vi "PC Code for Music Player.vi"() -> ()   [LabVIEW 2014]
uses:
  <vilib>/Utility/file.llb/Read From Spreadsheet File (I64).vi
panel:
  in  "stop":bool
  out "Debug Durations":i32[](array[numeric])
  out "Debug Notes":i32[](array[numeric])
  out "Durations":i32[](array[numeric])
  out "Notes":i32[](array[numeric])
  out "Full Music Array":i32[][](array[numeric])
  in  "Music File":path
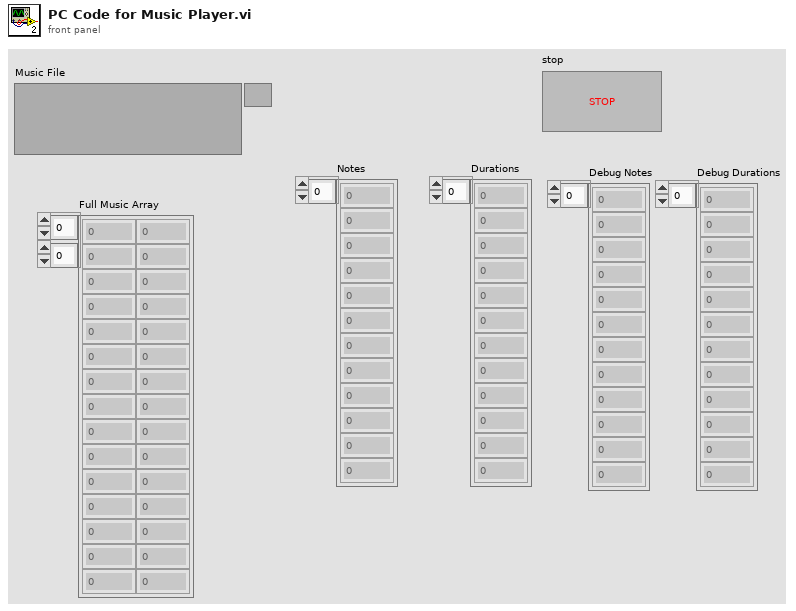
[diagram p1: front panel]
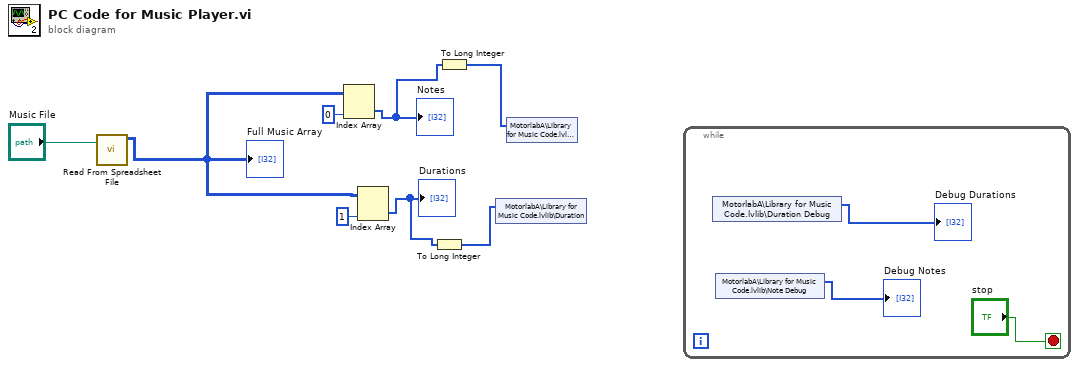
[diagram p0: block diagram]
diagram:
  n1 = call-poly <vilib>:"Read From Spreadsheet File.vi"("file path (dialog if empty)"="Music File") -> ("all rows"=w6:i64[][])  [unwired: 6 in, 4 out]
  "Full Music Array" <- w6
  n2 = Index Array(array=w6, index (col)=0 ("disabled index (col)")) -> (element=w4:i64[])  [unwired: 1 in]
  "Notes" <- w4
  n3 = Index Array(array=w6, index (col)=1 ("disabled index (col)")) -> (element=w2:i64[])  [unwired: 1 in]
  "Durations" <- w2
  n4 = To Long Integer(number=w2) -> (32bit integer=w1:i32[])
  n5 = To Long Integer(number=w4) -> (32bit integer=w3:i32[])
  n6 = shared-variable "MotorlabA\\Library for Music Code.lvlib\\Duration"(w1) -> ()  [unwired: 1 in, 1 out]
  n7 = shared-variable "MotorlabA\\Library for Music Code.lvlib\\Note"(w3) -> ()  [unwired: 1 in, 1 out]
  n8 = while {
    stop <- "stop" stop-if-true
    n9 = shared-variable "MotorlabA\\Library for Music Code.lvlib\\Duration Debug"() -> (→"Debug Durations":i32[])  [unwired: 1 in, 1 out]
    n10 = shared-variable "MotorlabA\\Library for Music Code.lvlib\\Note Debug"() -> (→"Debug Notes":i32[])  [unwired: 1 in, 1 out]
  }
